vi "TCP Send Command Respone.vi"(8 "error in (no error)":errorcluster, 10 "Response":string, 11 "connection ID":T1) -> (0 "error out":errorcluster, 3 "connection ID(dup)":T1)   [LabVIEW 2020, in "CSM-TCP-Router.lvlib"]
uses:
  CSM-TCP-Router.lvlib
  <vilib>/addons/_JKI.lib/_JKI_lib_TCP_Server.llb/TCP Server Connection Session ID Cluster.ctl
  tcp-msg type.ctl
  <userlib>/_NEVSTOP/Communicable State Machine(CSM)/AdvanceAPI/CSM - Make String Arguments Safe.vi
  <userlib>/_NEVSTOP/Communicable State Machine(CSM)/AdvanceAPI/CSM - Keywords.vi
  <userlib>/_NEVSTOP/Communicable State Machine(CSM)/Communicable State Machine.lvlib
  <vilib>/addons/_JKI.lib/_JKI_lib_TCP_Server.llb/JKI TCP Server.lvclass
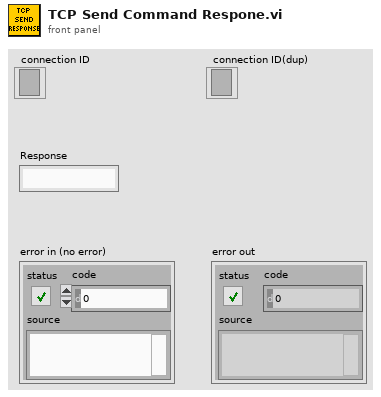
[diagram p1: front panel]
types:
  T1 = typedef "JKI TCP Server.lvclass/TCP Server Connection Session ID Cluster.ctl" = refnum<k5>
  T2 = typedef "CSM-TCP-Router.lvlib/tcp-msg type.ctl" = enum8{"info", "error", "cmd", "cmd-resp", "resp", "async-resp", "status", "interrupt"}
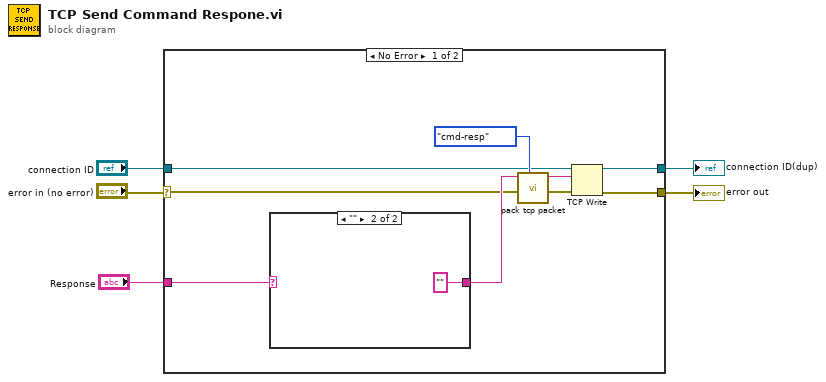
[diagram p0: block diagram]
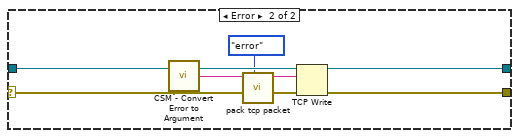
[diagram p3: hidden frame]
diagram:
  n1 = case shown="No Error" "error in (no error)" {
    selector: "error in (no error)" -> [w6 w16]
    tunnel: "connection ID" -> [w7 w22]
    tunnel: [w9 w21] -> w4
    tunnel: [w8 w19] -> w5
    tunnel: "Response" -> [w10 _]
    frame No Error {
      n2 = case shown="\"\"" w10 {
        selector: w10 -> [w14 _]
        tunnel: [w14 ""] -> w11
        frame Default {
        }
        frame "" {
        }
      }
      n3 = call "pack tcp packet.vi"("tcp-message-type"=tcp-msg_type."cmd-resp", "String"=w11) -> ("TCP Pack"=w12:string)  [unwired: 9 in]
      n4 = TCP Write(connection ID=w7, data in=w12, error in (no error)=w6) -> (connection ID out=w8:T1, error out=w9:errorcluster)  [unwired: 1 in, 1 out]
    }
    frame Error {
      n5 = call <userlib>:"CSM - Convert Error to Argument.vi"("Error"=w16) -> ("Argument"=w20:string)  [unwired: 4 in]
      n6 = call "pack tcp packet.vi"("tcp-message-type"=tcp-msg_type."error", "String"=w20) -> ("TCP Pack"=w18:string)  [unwired: 9 in]
      n7 = TCP Write(connection ID=w22, data in=w18, error in (no error)=w16) -> (connection ID out=w19:T1, error out=w21:errorcluster)  [unwired: 1 in, 1 out]
    }
  }
  "connection ID(dup)" <- w5
  "error out" <- w4
